vi "Debug Array.vi"(8 "error in (no error)":errorcluster, 11 "Priority Queue in":refnum<class "NI_Robotics_Priority Queue.lvclass">) -> (0 "error out":errorcluster, 2 "subarray":T1[](array[typedef]), 3 "Priority Queue out":refnum<class "NI_Robotics_Priority Queue.lvclass">)   [LabVIEW 2017, in "NI_Robotics_Priority Queue.lvclass"]
uses:
  <vilib>/robotics/Navigation/shared/Priority Queue/NI_Robotics_Priority Queue.lvclass
  <vilib>/robotics/Navigation/shared/Priority Queue/Open List Element.ctl
  <vilib>/robotics/Navigation/shared/MapNode/AbstractMapNode/NI_Robotics_AbstractMapNode.lvclass
  <vilib>/robotics/Navigation/shared/Priority Queue/NI_Robotics_Priority Queue.lvclass/NI_Robotics_Priority Queue.ctl
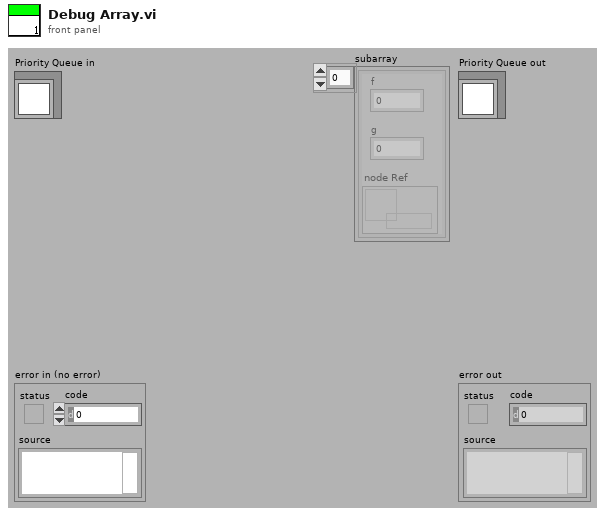
[diagram p1: front panel]
types:
  T1 = typedef "NI_Robotics_Priority Queue.lvclass/Open List Element.ctl" = cluster{"f":dbl, "g":dbl, "node Ref":refnum<data-value>}
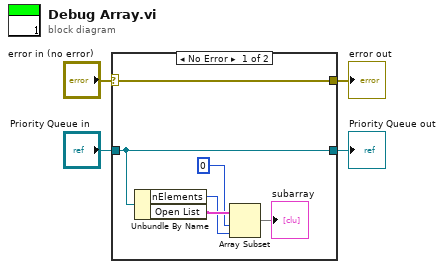
[diagram p0: block diagram]
diagram:
  n1 = case shown="No Error" "error in (no error)" {
    selector: "error in (no error)" -> [w10 w12]
    tunnel: [w10 w12] -> w3
    tunnel: [w9 w11] -> w1
    tunnel: "Priority Queue in" -> [w9 w11]
    frame No Error {
      n2 = Unbundle By Name(w9) -> ("nElements"=w7:i32, "Open List"=w8:T1[])
      n3 = Array Subset(array=w8, index=0, length=w7) -> (→"subarray":T1[])
    }
    frame Error {
    }
  }
  "error out" <- w3
  "Priority Queue out" <- w1
